vi "ziExample-DIO.vi"() -> ()   [LabVIEW 2009]
doc: "Control a Zurich instrument device via the LabOne Labview API. \nRequirements: Zurich Instruments MFLI, HF2 or UHFLI \nThe example streams the auxiliary digital input.\n\n© Zurich Instruments AG, www.zhinst.com"
uses:
  <instrlib>/Zurich Instruments LabOne/Public/Data/ziGetEventDIOSample.vi
  <instrlib>/Zurich Instruments LabOne/Zurich Instruments LabOne.lvlib
panel:
  out "DIO Out":T1
  out "Error Out":errorcluster
  in  "Address":string="DEV"
  out "Selected Device":string
  out "Unexpected Node":string[](array[string])
  in  "stop":bool=TRUE
  out "Timestamps":u64[](graph)=[1435629509284, 1435629939412, 1435630369530, 1435630799650, 1435631229770, 1435631659890, 1435632090010, 1435632520130, 1435632950248, 1435633380368, 1435633810486, 1435634240606, 1435634670726, 1435635100846, 1435635530966, 1435635961084, 1435636391204, 1435636821322, 1435637251442, 1435637681562, 1435638111682, 1435638541810, 1435638971928, 1435639402048, 1435639832168, 1435640262288]
  out "Digital Data":u32[](graph)=[3, 3, 3, 3, 3, 3, 3, 3, 3, 3, 3, 3, 3, 3, 3, 3, 3, 3, 3, 3, 3, 3, 3, 3, 3, 3]
  # "ziExample-DIO.vi\nRequirements: HF2LI, UHFLI and MFLI\nsee block diagram for VI description"
  # "Tested Instruments:\n- MFLI\n- HF2LI\n- UHFLI"
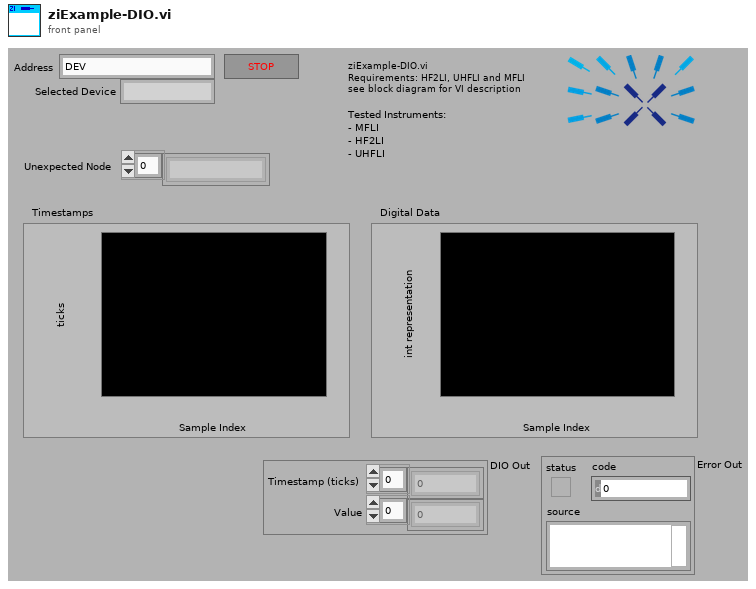
[diagram p1: front panel]
types:
  T1 = cluster{"Timestamp (ticks)":u64[], "Value":u32[]}
  T2 = typedef "Zurich Instruments LabOne.lvlib/ziTypeHandle.ctl" = cluster{"handleValid":bool, "Conn":u64, "Path Prefix":string, "Handle":u64, "Connected":bool, "Clockbase(s)":dbl}
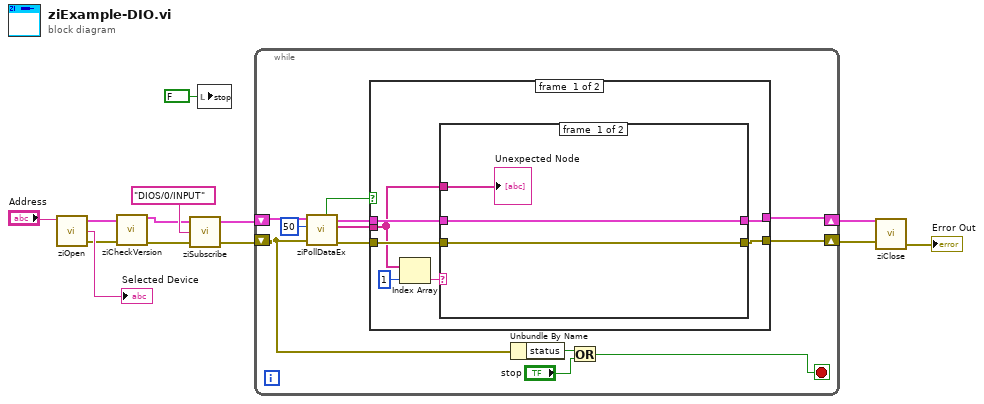
[diagram p0: block diagram]
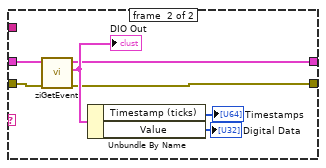
[diagram p2: hidden frame]
diagram:
  n1 = call <instrlib>:"ziOpen.vi"("Address"="Address") -> ("Error Out"=w3:errorcluster, "Selected Device"=→"Selected Device":string, "HandleOut"=w4:T2)  [unwired: 3 in]
  n2 = call <instrlib>:"ziCheckVersion.vi"("Handle In"=w4, "Error In"=w3) -> ("Handle Out"=w1:T2, "Error Out"=w2:errorcluster)  [unwired: 11 in, 1 out]
  n3 = call <instrlib>:"ziSubscribe.vi"("error in"=w2, "Path ()"="DIOS/0/INPUT", "Handle In"=w1) -> ("error out"=w11:errorcluster, "Handle Out"=w10:T2)  [unwired: 1 in]
  n4 = local write "stop"(FALSE ("stop")) -> ()
  n5 = while {
    shift-right: [w19] -> w12
    shift-left: w10 -> [w25]
    shift-right: [w18] -> w13
    shift-left: w11 -> [w15]
    stop <- w14 stop-if-true
    n6 = call <instrlib>:"ziPollDataEx.vi"("error in"=w15, "Timeout ms (50)"=50 ("TimeOut ms (50)"), "Handle In"=w25) -> ("error out"=w20:errorcluster, "PathArray"=w23:string[], "Handle Out"=w21:T2, "Timed Out"=w24:bool)  [unwired: 1 in, 4 out]
    n7 = case shown="False" w24 {
      tunnel: w23 -> [w26 _]
      tunnel: w21 -> [w32 w44]
      tunnel: w20 -> [w31 w43]
      tunnel: [w30 w44] -> w19
      tunnel: [w29 w43] -> w18
      frame #0 {
        n8 = Index Array(array=w26, index=1) -> (element=w27:string)
        n9 = case shown="\"DIOS\"" w27 {
          tunnel: w32 -> [w35 w42]
          tunnel: w31 -> [w34 w41]
          tunnel: [w35 w39] -> w30
          tunnel: [w34 w38] -> w29
          tunnel: w26 -> [w33 _]
          frame #0 {
            "Unexpected Node" <- w33
          }
          frame #1 {
            n10 = call-poly <instrlib>:"ziGetEvent.vi"("Error In"=w41, "Handle In"=w42) -> ("Error Out"=w38:errorcluster, "DIO Out"=w40:T1, "Handle Out"=w39:T2)  [unwired: 7 in]
            "DIO Out" <- w40
            n11 = Unbundle By Name(w40) -> ("Timestamp (ticks)"=→"Timestamps":u64[], "Value"=→"Digital Data":u32[])
          }
        }
      }
      frame #1 {
      }
    }
    n12 = Unbundle By Name(w15) -> ("status"=w17:bool)
    n13 = Or(x=w17, y="stop") -> (x .or. y?=w14:bool)
  }
  n14 = call <instrlib>:"ziClose.vi"("Error In"=w13, "Handle In"=w12) -> ("Error Out"=→"Error Out":errorcluster)  [unwired: 2 in, 1 out]
